vi "0x53_Cmd_write_table_parameter_data_(SubVI).vi"(9 "Parameters":T1 {"Шаг" min=0 step=4}, 10 "data":string, 11 "String in":string) -> (3 "String out":string)   [LabVIEW 2017, in "LV_Unicorn.lvlib"]
uses:
  LV_Unicorn.lvlib
panel:
  out "concatenated string 2":string
  out "concatenated string":string
  out "CRC-16-IBM":string
  out "length":i32
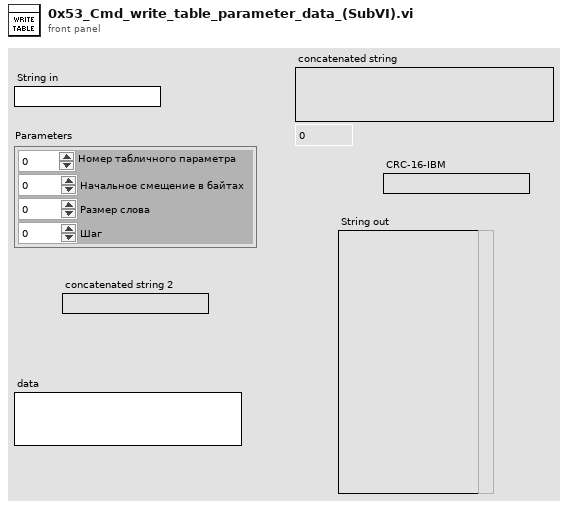
[diagram p1: front panel]
types:
  T1 = cluster{"Начальное смещение в байтах":i32, "Номер табличного параметра":i32, "Шаг":i32, "Размер слова":i32}
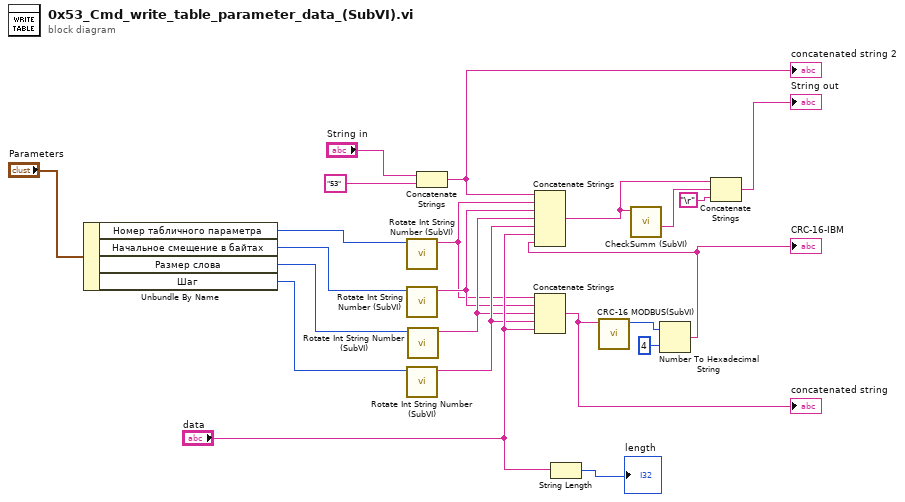
[diagram p0: block diagram]
diagram:
  n1 = Unbundle By Name("Parameters") -> ("Номер табличного параметра"=w16:i32, "Начальное смещение в байтах"=w15:i32, "Размер слова"=w12:i32, "Шаг"=w11:i32)
  n2 = call "Rotate Int String Number (SubVI).vi"("Int Number In"=w16) -> ("Orig String"=w2:string)  [unwired: 8 in, 2 out]
  n3 = call "Rotate Int String Number (SubVI).vi"("Int Number In"=w15) -> ("Orig String"=w4:string)  [unwired: 8 in, 2 out]
  n4 = call "Rotate Int String Number (SubVI).vi"("Int Number In"=w11) -> ("Orig String"=w6:string)  [unwired: 8 in, 2 out]
  n5 = call "Rotate Int String Number (SubVI).vi"("Int Number In"=w12) -> ("Orig String"=w5:string)  [unwired: 8 in, 2 out]
  n6 = Concatenate Strings("String in", "53" ("string")) -> (w20:string)
  "concatenated string 2" <- w20
  n7 = Concatenate Strings(w2, w4, w5, w6, "data") -> (w1:string)
  "concatenated string" <- w1
  n8 = String Length(string="data") -> (length=→"length":i32)
  n9 = call "CRC-16 MODBUS(SubVI).vi"("string in"=w1) -> ("CRC-16-IBM"=w9:u16)  [unwired: 10 in]
  n10 = Number To Hexadecimal String(1:i16 4 ("width (-)"), 2:w9) -> (0:w8:string)
  "CRC-16-IBM" <- w8
  n11 = Concatenate Strings(w20, w2, w4, w5, w6, "data", w8) -> (w3:string)
  n12 = call "CheckSumm (SubVI).vi"("Input String"=w3) -> ("CheckSumm"=w17:string)  [unwired: 7 in, 3 out]
  n13 = Concatenate Strings(w3, w17, "\r") -> (→"String out":string)
